vi "Update UI.vi"(0 "Stage Controller in":refnum<class "TripleAxisStageController.lvclass">, 5 "DataExchange":T1, 11 "error in (no error)":errorcluster) -> (4 "Stage Controller out":refnum<class "TripleAxisStageController.lvclass">, 15 "error out":errorcluster)   [LabVIEW 2020, in "TripleAxisStageController.lvlib" / "TripleAxisStageController.lvclass"]
uses:
  TripleAxisStageController.lvclass
  Model/Hardware Abstraction Layer/Component/Device/Device/DataExchange.ctl
  TripleAxisStageController.lvclass/TripleAxisStageController.ctl
  Interface/DataListener/DataListener.lvclass
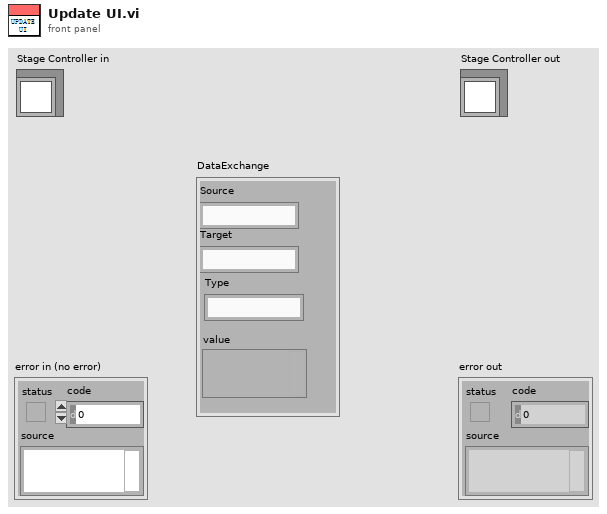
[diagram p1: front panel]
types:
  T1 = typedef "DataListener.lvclass/DataExchange.ctl" = cluster{"Source":string, "Target":string, "Type":string, "value":variant}
  T2 = cluster{"Stage X Position":dbl, "Stage Y Position":dbl, "Stage Z Position":dbl}
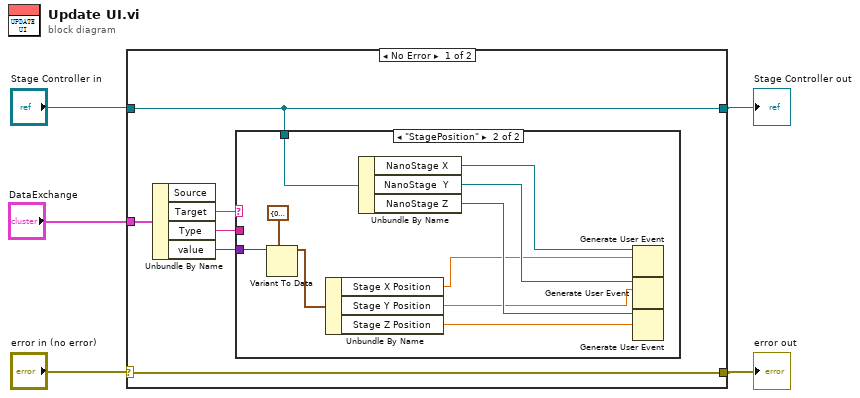
[diagram p0: block diagram]
diagram:
  n1 = case shown="No Error" "error in (no error)" {
    selector: "error in (no error)" -> [w11 w23]
    tunnel: [w11 w23] -> w2
    tunnel: [w6 w22] -> w3
    tunnel: "Stage Controller in" -> [w6 w22]
    tunnel: "DataExchange" -> [w10 _]
    frame No Error {
      n2 = Unbundle By Name(w10) -> ("Target"=w7:string, "Type"=w8:string, "value"=w9:variant)  [unwired: 1 out]
      n3 = case shown="\"StagePosition\"" w7 {
        tunnel: w9 -> [_ w21]
        tunnel: w8 -> [_ _]
        tunnel: w6 -> [_ w20]
        frame "False", Default {
        }
        frame "StagePosition" {
          n4 = Variant To Data(type=T2 {"Stage X Position"=0.0, "Stage Y Position"=0.0, "Stage Z Position"=0.0} ("Cluster"), Variant=w21) -> (data=w15:T2)  [unwired: 1 in, 1 out]
          n5 = Unbundle By Name(w15) -> ("Stage X Position"=w14:dbl, "Stage Y Position"=w13:dbl, "Stage Z Position"=w12:dbl)
          n6 = Unbundle By Name(w20) -> ("NanoStage X"=w19:refnum<user-event>, "NanoStage  Y"=w17:refnum<user-event>, "NanoStage Z"=w16:refnum<user-event>)
          n7 = Generate User Event(user event=w19, event data cluster=w14) -> ()  [unwired: 2 in, 2 out]
          n8 = Generate User Event(user event=w17, event data cluster=w13) -> ()  [unwired: 2 in, 2 out]
          n9 = Generate User Event(user event=w16, event data cluster=w12) -> ()  [unwired: 2 in, 2 out]
        }
      }
    }
    frame Error {
    }
  }
  "error out" <- w2
  "Stage Controller out" <- w3
